vi "Server.Settings.vi"(6 "Action":enum8{"Get", "Set"}(ring), 8 "error in (no error)":errorcluster, 10 "Client Settings In":T1, 11 "Parent Ref in":T2 format="%.0x") -> (0 "error out":errorcluster, 2 "Client Settings Out":T1, 3 "Item Ref out":T2 format="%.0x")   [LabVIEW 2020, in "gRPC Data Server Shared.lvlib"]
uses:
  gRPC Data Server Shared.lvlib
  Compiled.Settings.ctl
  <vilib>/NI VeriStand/Custom Device API/Custom Device Item Ref.ctl
  Constants.vi
  <vilib>/NI VeriStand/Custom Device API/Set Item Property (String).vi
  <vilib>/NI VeriStand/Custom Device API/Set Item Property (Boolean).vi
  <vilib>/NI VeriStand/Custom Device API/Set Item Property (Path).vi
  <vilib>/NI VeriStand/Custom Device API/Set Item Property (String Array).vi
  <vilib>/NI VeriStand/Custom Device API/Get Item Property (String).vi
  <vilib>/NI VeriStand/Custom Device API/Get Item Property (Boolean).vi
  <vilib>/NI VeriStand/Custom Device API/Get Item Property (Path).vi
  <vilib>/NI VeriStand/Custom Device API/Get Item Property (String Array).vi
  <vilib>/NI VeriStand/Custom Device API/Custom Device API.lvlib
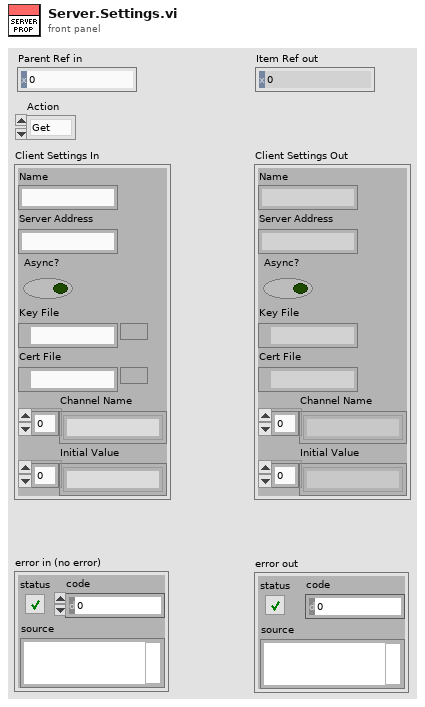
[diagram p1: front panel]
types:
  T1 = typedef "gRPC Data Server Shared.lvlib/Compiled.Settings.ctl" = cluster{"Name":string, "Server Address":string, "Async?":bool, "Key File":path, "Cert File":path, "Channel Name":string[], "Initial Value":string[]}
  T2 = typedef "Custom Device API.lvlib/Custom Device Item Ref.ctl" = u64
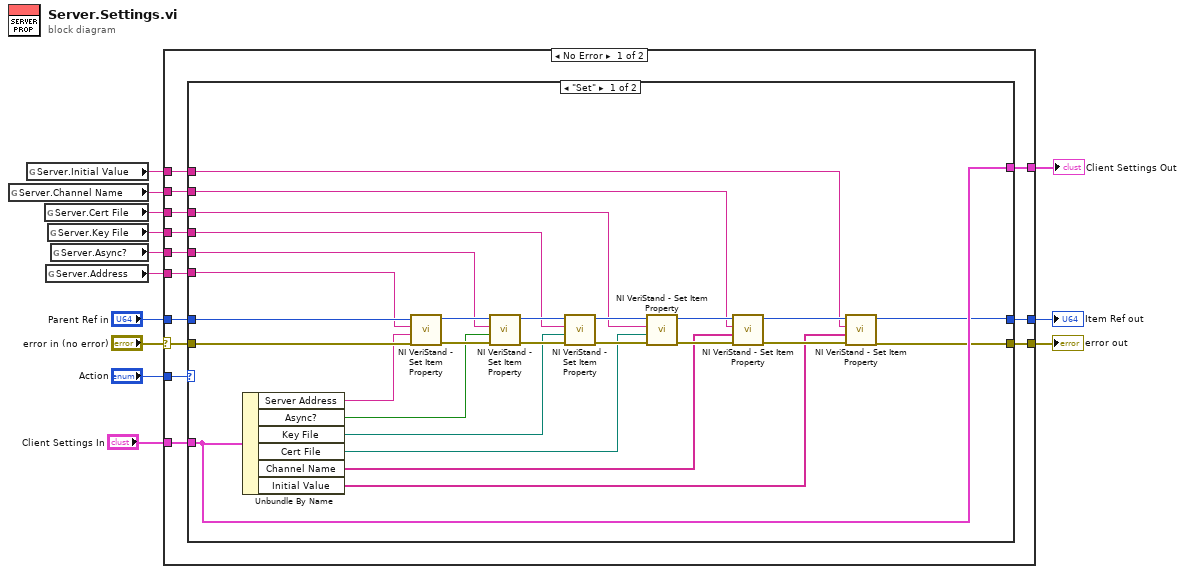
[diagram p0: block diagram]
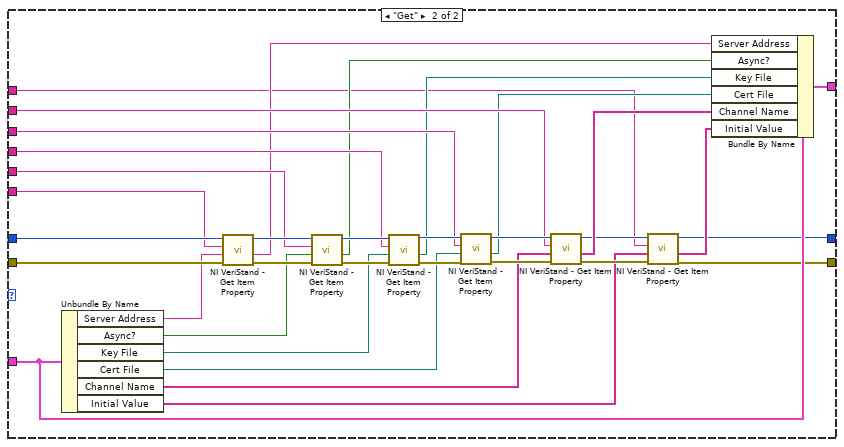
[diagram p2: hidden frame]
diagram:
  n1 = global read "Constants.vi" "Server.Channel Name"() -> (w2:string)
  n2 = global read "Constants.vi" "Server.Initial Value"() -> (w1:string)
  n3 = global read "Constants.vi" "Server.Cert File"() -> (w3:string)
  n4 = global read "Constants.vi" "Server.Address"() -> (w6:string)
  n5 = global read "Constants.vi" "Server.Key File"() -> (w4:string)
  n6 = global read "Constants.vi" "Server.Async?"() -> (w5:string)
  n7 = case shown="No Error" "error in (no error)" {
    selector: "error in (no error)" -> [w22 w90]
    tunnel: "Parent Ref in" -> [w26 w89]
    tunnel: "Client Settings In" -> [w25 w88]
    tunnel: [w24 w90] -> w11
    tunnel: [w23 w89] -> w10
    tunnel: "Action" -> [w21 _]
    tunnel: [w20 w88] -> w7
    tunnel: w6 -> [w19 _]
    tunnel: w4 -> [w18 _]
    tunnel: w5 -> [w17 _]
    tunnel: w3 -> [w16 _]
    tunnel: w2 -> [w15 _]
    tunnel: w1 -> [w14 _]
    frame No Error {
      n8 = case shown="\"Set\"" w21 {
        tunnel: w26 -> [w52 w87]
        tunnel: w25 -> [w53 w78]
        tunnel: [w30 w54] -> w24
        tunnel: [w31 w55] -> w23
        tunnel: w19 -> [w46 w82]
        tunnel: w17 -> [w45 w81]
        tunnel: w18 -> [w44 w80]
        tunnel: w22 -> [w51 w79]
        tunnel: [w53 w77] -> w20
        tunnel: w16 -> [w39 w73]
        tunnel: w15 -> [w36 w70]
        tunnel: w14 -> [w28 w57]
        frame "Set" {
          n9 = Unbundle By Name(w53) -> ("Server Address"=w43:string, "Async?"=w42:bool, "Key File"=w35:path, "Cert File"=w34:path, "Channel Name"=w33:string[], "Initial Value"=w27:string[])
          n10 = call-poly <vilib>:"NI VeriStand - Set Item Property.vi"("error in (no error)"=w51, "Value"=w43, "Property Name"=w46, "Item Ref in"=w52) -> ("error out"=w49:errorcluster, "Item Ref out"=w50:T2)  [unwired: 5 in, 1 out]
          n11 = call-poly <vilib>:"NI VeriStand - Set Item Property.vi"("error in (no error)"=w49, "Value"=w42, "Property Name"=w45, "Item Ref in"=w50) -> ("error out"=w47:errorcluster, "Item Ref out"=w48:T2)  [unwired: 5 in, 1 out]
          n12 = call-poly <vilib>:"NI VeriStand - Set Item Property.vi"("error in (no error)"=w47, "Value"=w35, "Property Name"=w44, "Item Ref in"=w48) -> ("error out"=w40:errorcluster, "Item Ref out"=w41:T2)  [unwired: 5 in, 1 out]
          n13 = call-poly <vilib>:"NI VeriStand - Set Item Property.vi"("error in (no error)"=w40, "Value"=w34, "Property Name"=w39, "Item Ref in"=w41) -> ("error out"=w37:errorcluster, "Item Ref out"=w38:T2)  [unwired: 5 in, 1 out]
          n14 = call-poly <vilib>:"NI VeriStand - Set Item Property.vi"("error in (no error)"=w37, "Value"=w33, "Property Name"=w36, "Item Ref in"=w38) -> ("error out"=w29:errorcluster, "Item Ref out"=w32:T2)  [unwired: 5 in, 1 out]
          n15 = call-poly <vilib>:"NI VeriStand - Set Item Property.vi"("error in (no error)"=w29, "Value"=w27, "Property Name"=w28, "Item Ref in"=w32) -> ("error out"=w30:errorcluster, "Item Ref out"=w31:T2)  [unwired: 5 in, 1 out]
        }
        frame "Get" {
          n16 = Unbundle By Name(w78) -> ("Server Address"=w76:string, "Async?"=w69:bool, "Key File"=w68:path, "Cert File"=w67:path, "Channel Name"=w66:string[], "Initial Value"=w56:string[])
          n17 = call-poly <vilib>:"NI VeriStand - Get Item Property.vi"("error in (no error)"=w79, "Default Value"=w76, "Property Name"=w82, "Item Ref in"=w87) -> ("error out"=w85:errorcluster, "Value"=w65:string, "Item Ref out"=w86:T2)  [unwired: 4 in, 1 out]
          n18 = call-poly <vilib>:"NI VeriStand - Get Item Property.vi"("error in (no error)"=w85, "Default Value"=w69, "Property Name"=w81, "Item Ref in"=w86) -> ("error out"=w84:errorcluster, "Value"=w64:bool, "Item Ref out"=w83:T2)  [unwired: 4 in, 1 out]
          n19 = call-poly <vilib>:"NI VeriStand - Get Item Property.vi"("error in (no error)"=w84, "Default Value"=w68, "Property Name"=w80, "Item Ref in"=w83) -> ("error out"=w74:errorcluster, "Value"=w63:path, "Item Ref out"=w75:T2)  [unwired: 4 in, 1 out]
          n20 = call-poly <vilib>:"NI VeriStand - Get Item Property.vi"("error in (no error)"=w74, "Default Value"=w67, "Property Name"=w73, "Item Ref in"=w75) -> ("error out"=w71:errorcluster, "Value"=w62:path, "Item Ref out"=w72:T2)  [unwired: 4 in, 1 out]
          n21 = call-poly <vilib>:"NI VeriStand - Get Item Property.vi"("error in (no error)"=w71, "Default Value"=w66, "Property Name"=w70, "Item Ref in"=w72) -> ("error out"=w59:errorcluster, "Value"=w61:string[], "Item Ref out"=w60:T2)  [unwired: 4 in, 1 out]
          n22 = call-poly <vilib>:"NI VeriStand - Get Item Property.vi"("error in (no error)"=w59, "Default Value"=w56, "Property Name"=w57, "Item Ref in"=w60) -> ("error out"=w54:errorcluster, "Value"=w58:string[], "Item Ref out"=w55:T2)  [unwired: 4 in, 1 out]
          n23 = Bundle By Name(cluster=w78, "Server Address"=w65, "Async?"=w64, "Key File"=w63, "Cert File"=w62, "Channel Name"=w61, "Initial Value"=w58) -> (w77:T1)
        }
      }
    }
    frame Error {
    }
  }
  "Item Ref out" <- w10
  "error out" <- w11
  "Client Settings Out" <- w7
